vi "add_bool_roslv.vi"   [LabVIEW 2014]
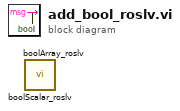
[diagram p0: block diagram]
diagram:
  n1 = call "boolScalar_roslv.vi"() -> ()  [unwired: 5 in, 1 out]
  n2 = call "boolArray_roslv.vi"() -> ()  [unwired: 5 in, 1 out]
